vi "SMU Switch Handshaking - LV code improvements - Streaming2.vi"(8 "error in":errorcluster, 10 "gRPCid":T1, 11 "file path (use dialog)":path=path "C:/Users/IES/Desktop/jsontestfile.json") -> (0 "error out":errorcluster, 3 "Elapsed Time":u32)   [LabVIEW 2019]
uses:
  labview-grpc-query-server/VIs/MeasurementServer_gRPCid.ctl
  <instrlib>/niDCPower/nidcpower.llb/niDCPower Send Software Edge Trigger - Signal.ctl
  labview-grpc-query-server/VIs/MeasurementServer_FourProbeRawData.ctl
  labview-grpc-query-server/VIs/MeasurementServer_ErrorOutData.ctl
  <instrlib>/niDCPower/nidcpower.llb/niDCPower Configure Software Edge Start Trigger.vi
  <instrlib>/niDCPower/nidcpower.llb/niDCPower Configure Software Edge Sequence Advance Trigger.vi
  labview-grpc-query-server/VIs/labview-grpc-measurement-server.lvlib
  SupportVIs.lvlib
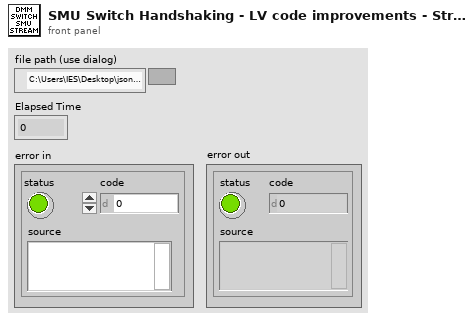
[diagram p1: front panel]
types:
  T1 = typedef "labview-grpc-measurement-server.lvlib/MeasurementServer_gRPCid.ctl" = u64
  T2 = typedef "niDCPower Send Software Edge Trigger - Signal.ctl" = i32
  T3 = typedef "JSONCluster.ctl" = cluster{"SMUResourceName":string, "SMUChannels":string, "SMUSourceMode_Sequence":i32, "SMUOutputFunction_DCCurrent":i32, "SMUSourceTransientResponse_Fast":i32, "SMUCurrent":dbl, "SMUCurrentLevelRange":dbl, "SMUMeasurementSense_Local":i32, "SMUMeasurementApertureTime":dbl, "SMUSourceAdvancedSourceDelay":dbl, "SMUVoltage":dbl, "SMUSourceAdvancedSequenceLoopCount":i32, "SMUMeasurementAdvancedDCNoiseRejection_Normal":i32, "SMUSequenceName":string, "SMUStep1_Source_DCCurrent_CurrentLevel":i32, "SMUStep2_Measurement_ApertureTime":i32, "SMUStep3_Source_Advanced_SourceDelay":i32, "SMUSequenceNumberOfSteps":i32, "SMUTriggerFromSwitch_StartDigitalEdge":string, "SMUTriggerFromSwitch_SequenceAdvanceDigitalEdge":string, "SMUTriggerToDMM_SourceCompleteEvent":i32, "SMUTriggerToDMM_SourceCompleteEvent_Value":string, "SMUTriggerToSwitch_SequenceIterationCompleteEvent":i32, "SMUTriggerToDMM_SequenceIterationCompleteEvent_Value":string, "Switch1ResourceName":string, "Switch1Topology":string, "Switch1ScanList":string, "Switch2ResourceName":string, "Switch2Topology":string, "Switch2ScanList":string, "DMMResourceName":string, "DMMFunction_DCVolts":i32, "DMMResolution":dbl, "DMMRange":dbl, "DMMTriggerSource_TTL2":i32, "DMMTriggerSlope_RisingEdge":i32, "DMMSampleTrigger_TTL2":i32, "DMMSampleCount":i32, "DMMSampleTriggerSlope_RisingEdge":i32, "DMMApertureTimeUnits_Seconds":i32, "DMMApertureTime":dbl, "DMMNumberOfAverages":i32, "DMMAutoZero_Off":i32, "DMMADCCalibration_Off":i32, "DMMSettleTime":dbl, "DMMControlAction_Commit":i32, "ApplicationNumberOfWeldChannels":i32}
  T4 = typedef "labview-grpc-measurement-server.lvlib/MeasurementServer_ErrorOutData.ctl" = cluster{"ErrorCode":i32, "ErrorMessage":string}
  T5 = typedef "labview-grpc-measurement-server.lvlib/MeasurementServer_FourProbeRawData.ctl" = cluster{"Positive Voltage":sgl, "Positive Current":sgl, "Negative Voltage":sgl, "Negative Current":sgl, "Impedance":sgl, "ErrorOutData":T4}
  T6 = typedef "niDMM Acquisition State.ctl" = enum16{"Running", "Finished with Backlog", "Finished with no Backlog", "Paused", "No acquisition in progress"}
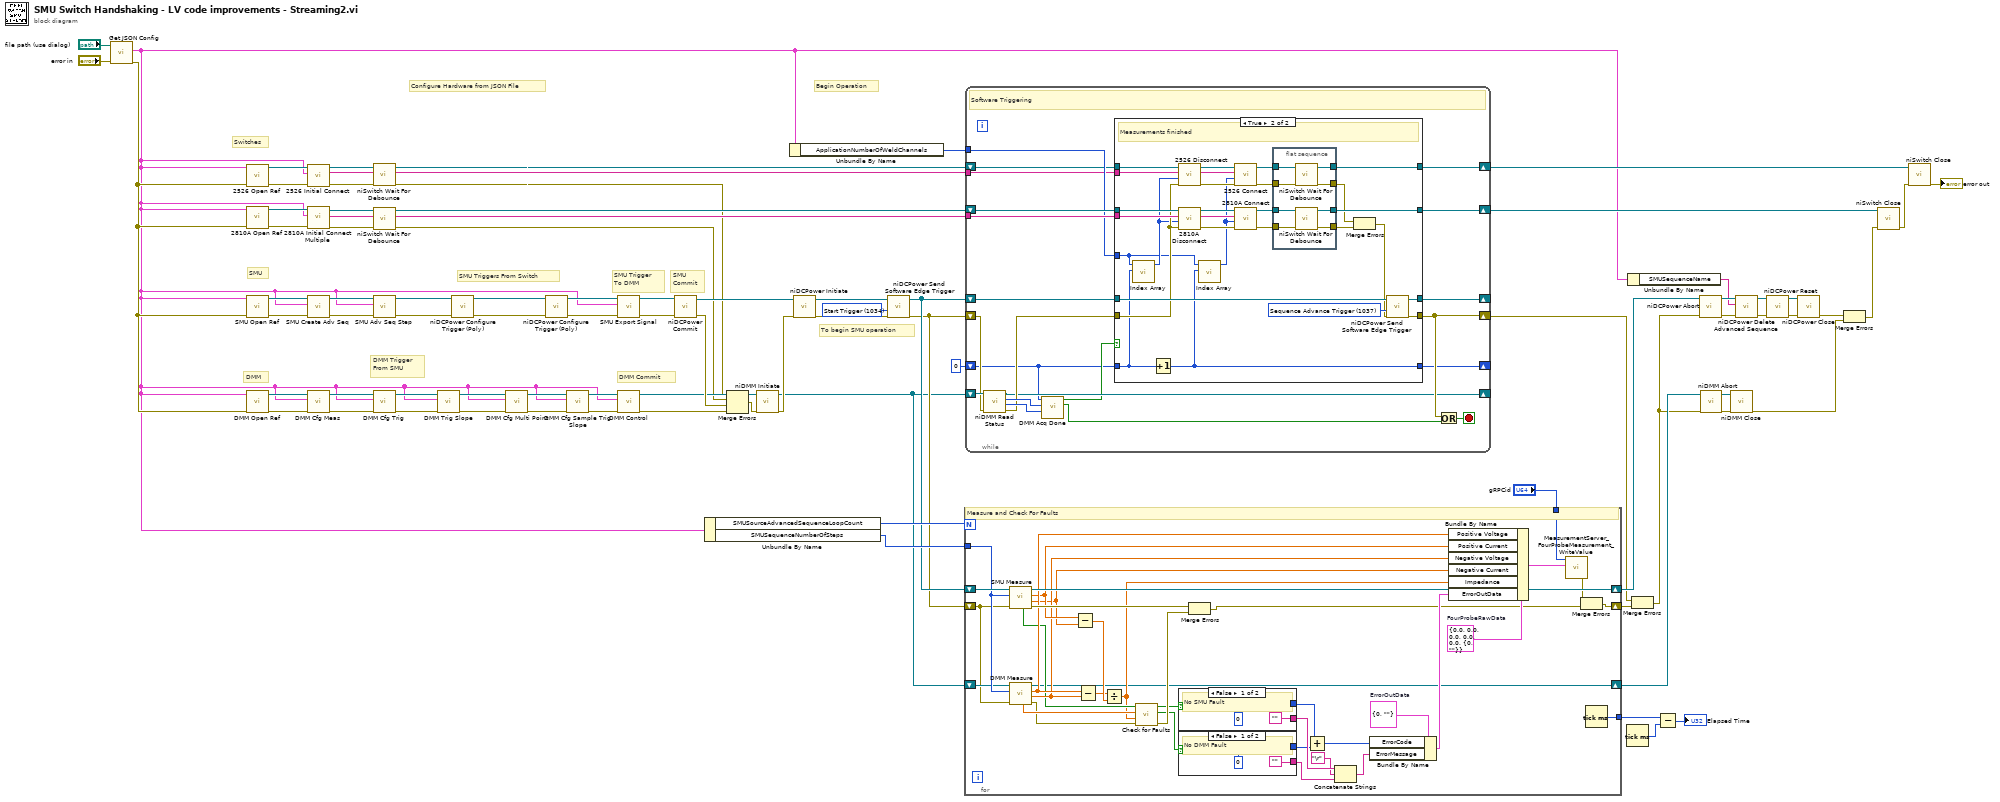
[diagram p0: block diagram]
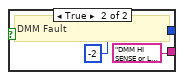
[diagram p3: hidden frame]
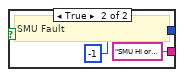
[diagram p4: hidden frame]
diagram:
  w35 = T2 1034 items=["Start Trigger"=1034, "Source Trigger"=1035, "Measure Trigger"=1036, "Sequence Advance Trigger"=1037, "Pulse Trigger"=1053] ("signal")
  # "SMU\nCommit"
  # "DMM Commit"
  # "Begin Operation"
  # "Configure Hardware from JSON File"
  # "DMM"
  # "SMU"
  # "Switches"
  # "To begin SMU operation"
  # "DMM Trigger\nFrom SMU"
  # "SMU Trigger \nTo DMM"
  # "SMU Triggers From Switch"
  n1 = call "Get JSON Config.vi"("error in (no error)"="error in", "JSON Configuration File (.json)"="file path (use dialog)") -> ("error out"=w9:errorcluster, "JSONCluster"=w2:T3)  [unwired: 6 in, 2 out]
  n2 = call "2526 Open Ref.vi"("error in"=w9, "JSONCluster"=w2) -> ("error out"=w21:errorcluster, "IVI Refnum out"=w22:refnum<k15>)  [unwired: 8 in]
  n3 = call "2810A Open Ref.vi"("error in"=w9, "JSONCluster"=w2) -> ("error out"=w28:errorcluster, "IVI Refnum out"=w29:refnum<k15>)  [unwired: 8 in]
  n4 = call "SMU Open Ref.vi"("error in (no error)"=w9, "JSONCluster"=w2) -> ("error out"=w82:errorcluster, "IVI Refnum out"=w83:refnum<k15>)  [unwired: 8 in]
  n5 = call "DMM Open Ref.vi"("error in"=w9, "JSONCluster"=w2) -> ("error out"=w55:errorcluster, "IVI Refnum out"=w54:refnum<k15>)  [unwired: 8 in]
  n6 = call "2526 Initial Connect.vi"("error in (no error)"=w21, "JSONCluster"=w2, "IVI Refnum in"=w22) -> ("error out"=w19:errorcluster, "2525 Scan List Channels"=w15:string[], "IVI Refnum out"=w20:refnum<k15>)  [unwired: 6 in]
  n7 = call "2810A Initial Connect Multiple.vi"("error in (no error)"=w28, "JSONCluster"=w2, "IVI Refnum in"=w29) -> ("error out"=w25:errorcluster, "Array"=w27:string[], "IVI Refnum out"=w26:refnum<k15>)  [unwired: 6 in]
  n8 = call "SMU Create Adv Seq.vi"("error in (no error)"=w82, "JSONCluster"=w2, "IVI Refnum in"=w83) -> ("error out"=w70:errorcluster, "IVI Refnum out"=w71:refnum<k15>)  [unwired: 7 in]
  n9 = call "DMM Cfg Meas.vi"("error in (no error)"=w55, "JSONCluster"=w2, "IVI Refnum in"=w54) -> ("error out"=w59:errorcluster, "IVI Refnum out"=w58:refnum<k15>)  [unwired: 7 in]
  n10 = call <instrlib>:"niSwitch Wait For Debounce.vi"("error in (no error)"=w19, "instrument handle"=w20) -> ("error out"=w17:errorcluster, "instrument handle out"=w16:refnum<k15>)  [unwired: 8 in]
  n11 = call <instrlib>:"niSwitch Wait For Debounce.vi"("error in (no error)"=w25, "instrument handle"=w26) -> ("error out"=w24:errorcluster, "instrument handle out"=w23:refnum<k15>)  [unwired: 8 in]
  n12 = call "SMU Adv Seq Step.vi"("error in (no error)"=w70, "JSONCluster"=w2, "IVI Refnum in"=w71) -> ("error out"=w68:errorcluster, "IVI Refnum out"=w69:refnum<k15>)  [unwired: 7 in]
  n13 = call "DMM Cfg Trig.vi"("error in (no error)"=w59, "JSONCluster"=w2, "IVI Refnum in"=w58) -> ("error out"=w61:errorcluster, "IVI Refnum out"=w60:refnum<k15>)  [unwired: 7 in]
  n14 = call "DMM Trig Slope.vi"("error in (no error)"=w61, "JSONCluster"=w2, "IVI Refnum in"=w60) -> ("error out"=w63:errorcluster, "IVI Refnum out"=w62:refnum<k15>)  [unwired: 7 in]
  n15 = call-poly <instrlib>:"niDCPower Configure Trigger (Poly).vi"("error in (no error)"=w68, "instrument handle"=w69) -> ("error out"=w79:errorcluster, "instrument handle out"=w80:refnum<k15>)  [unwired: 8 in]
  n16 = call "DMM Cfg Multi Point.vi"("error in (no error)"=w63, "JSONCluster"=w2, "IVI Refnum in"=w62) -> ("error out"=w65:errorcluster, "IVI Refnum out"=w64:refnum<k15>)  [unwired: 7 in]
  n17 = call-poly <instrlib>:"niDCPower Configure Trigger (Poly).vi"("error in (no error)"=w79, "instrument handle"=w80) -> ("error out"=w42:errorcluster, "instrument handle out"=w43:refnum<k15>)  [unwired: 8 in]
  n18 = call "DMM Cfg Sample Trig Slope.vi"("error in (no error)"=w65, "JSONCluster"=w2, "IVI Refnum in"=w64) -> ("error out"=w47:errorcluster, "IVI Refnum out"=w48:refnum<k15>)  [unwired: 7 in]
  n19 = call "SMU Export Signal.vi"("error in (no error)"=w42, "JSONCluster"=w2, "IVI Refnum in"=w43) -> ("error out"=w66:errorcluster, "IVI Refnum out"=w67:refnum<k15>)  [unwired: 7 in]
  n20 = call "DMM Control.vi"("error in (no error)"=w47, "JSONCluster"=w2, "IVI Refnum in"=w48) -> ("error out"=w52:errorcluster, "IVI Refnum out"=w49:refnum<k15>)  [unwired: 7 in]
  n21 = call <instrlib>:"niDCPower Commit.vi"("error in (no error)"=w66, "instrument handle"=w67) -> ("error out"=w53:errorcluster, "instrument handle out"=w50:refnum<k15>)  [unwired: 8 in]
  n22 = Unbundle By Name(w2) -> ("SMUSourceAdvancedSequenceLoopCount"=w38:i32, "SMUSequenceNumberOfSteps"=w37:i32)
  n23 = Merge Errors(w17, w24, w53, w52) -> (w51:errorcluster)
  n24 = call <instrlib>:"niDMM Initiate.vi"("error in (no error)"=w51, "instrument handle"=w49) -> ("error out"=w18:errorcluster, "instrument handle out"=w3:refnum<k15>)  [unwired: 8 in]
  n25 = Unbundle By Name(w2) -> ("ApplicationNumberOfWeldChannels"=w31:i32)
  n26 = call <instrlib>:"niDCPower Initiate.vi"("error in (no error)"=w18, "instrument handle"=w50) -> ("error out"=w30:errorcluster, "instrument handle out"=w36:refnum<k15>)  [unwired: 8 in]
  n27 = call <instrlib>:"niDCPower Send Software Edge Trigger.vi"("error in (no error)"=w30, "signal"=w35, "instrument handle"=w36) -> ("error out"=w4:errorcluster, "instrument handle out"=w5:refnum<k15>)  [unwired: 7 in]
  n28 = for {
    N: w38 -> [_]
    tunnel: w37 -> [w91]
    shift-right: [w89] -> w7
    shift-left: w4 -> [w87]
    shift-right: [w119] -> w81
    shift-left: w5 -> [w92]
    shift-right: [w85] -> w44
    shift-left: w3 -> [w88]
    tunnel: [w96] -> w10
    tunnel: "gRPCid" -> [w95]
    w97 = T4 {"ErrorCode"=0, "ErrorMessage"=""}  # ErrorOutData
    w94 = T5 {"Positive Voltage"=0.0, "Positive Current"=0.0, "Negative Voltage"=0.0, "Negative Current"=0.0, "Impedance"=0.0, "ErrorOutData"={"ErrorCode"=0, "ErrorMessage"=""}}  # FourProbeRawData
    # "Measure and Check For Faults"
    n29 = call "SMU Measure.vi"("error in (no error)"=w87, "SMUSequenceNumberOfSteps"=w91, "IVI Refnum in"=w92) -> ("error out"=w118:errorcluster, "Numeric"=w111:dbl, "Numeric 2"=w113:dbl, "IVI Refnum out"=w119:refnum<k15>, "in compliance"=w100:bool[])  [unwired: 4 in]
    n30 = call "DMM Measure.vi"("error in (no error)"=w87, "SMUSequenceNumberOfSteps"=w91, "IVI Refnum in"=w88) -> ("error out"=w86:errorcluster, "Numeric"=w112:dbl, "Numeric 2"=w114:dbl, "IVI Refnum out"=w85:refnum<k15>, "Measurements"=w99:dbl[])  [unwired: 4 in]
    n31 = Subtract(x=w113, y=w111) -> (x-y=w116:dbl)
    n32 = Subtract(x=w114, y=w112) -> (x-y=w115:dbl)
    n33 = Divide(x=w115, y=w116) -> (x/y=w98:dbl)
    n34 = call "Check for Faults.vi"("Error In"=w86, "Resistance In"=w98, "dmm voltage measurements"=w99, "in compliance"=w100) -> ("Error Out"=w117:errorcluster, "DMM Fault"=w104:bool, "SMU Fault"=w108:bool)  [unwired: 4 in, 1 out]
    n35 = case shown="False" w108 {
      tunnel: ["" "SMU HI or LO lead disconnected\n- SMU in compliance\n- SMU Fault = True"] -> w107
      tunnel: [0 -1] -> w105
      frame False {
        # "No SMU Fault"
      }
      frame True {
        # "SMU Fault"
      }
    }
    n36 = case shown="False" w104 {
      tunnel: ["" "DMM HI SENSE or LO SENSE lead disconnected\n- DMM measures NaN, or \n- DMM overrange warning, or\n- DMM voltage > 50uV "] -> w102
      tunnel: [0 -2] -> w101
      frame False {
        # "No DMM Fault"
      }
      frame True {
        # "DMM Fault"
      }
    }
    n37 = Merge Errors(w118, w117) -> (w84:errorcluster)
    n38 = Add(x=w105, y=w101) -> (x+y=w109:i32)
    n39 = Concatenate Strings(w107, "\r", w102) -> (w106:string)
    n40 = Bundle By Name(cluster=w97, "ErrorCode"=w109, "ErrorMessage"=w106) -> (w110:T4)
    n41 = Bundle By Name(cluster=w94, "Positive Voltage"=w114, "Positive Current"=w113, "Negative Voltage"=w112, "Negative Current"=w111, "Impedance"=w98, "ErrorOutData"=w110) -> (w93:T5)
    n42 = call "MeasurementServer_FourProbeMeasurement_WriteValue.vi"("gRPCid"=w95, "FourProbeRawData"=w93) -> ("error out"=w90:errorcluster)  [unwired: 8 in]
    n43 = Merge Errors(w90, w84) -> (w89:errorcluster)
    n44 = Tick Count (ms)() -> (millisecond timer value=w96:u32)
  }
  n45 = while {
    shift-right: [w148] -> _
    shift-left: w5 -> [w143]
    shift-right: [w146] -> w1
    shift-left: w4 -> [w133]
    shift-right: [w144] -> w32
    shift-left: w23 -> [w145]
    shift-right: [w131] -> _
    shift-left: w3 -> [w134]
    shift-right: [w142] -> _
    shift-left: 0 ("Backlog") -> [w128]
    tunnel: w27 -> [w141]
    tunnel: w31 -> [w140]
    shift-right: [w138] -> w14
    shift-left: w16 -> [w139]
    tunnel: w15 -> [w137]
    stop <- w147 stop-if-true
    # "Software Triggering"
    n46 = call <instrlib>:"niDMM Read Status.vi"("error in (no error)"=w133, "instrument handle"=w134) -> ("error out"=w132:errorcluster, "Acquisition State"=w135:T6, "Backlog"=w136:i32, "instrument handle out"=w131:refnum<k15>)  [unwired: 6 in]
    n47 = call "DMM Acq Done.vi"("Acquisition State"=w135, "Backlog"=w136, "Channel Index"=w128) -> ("Finished with Backlog?"=w129:bool, "Sequence Acquision Finished?"=w130:bool)  [unwired: 7 in]
    n48 = case shown="True" w130 {
      tunnel: w132 -> [w152 w162]
      tunnel: [w153 w180] -> w148
      tunnel: [w152 w179] -> w146
      tunnel: w143 -> [w153 w176]
      tunnel: w145 -> [w151 w175]
      tunnel: [w151 w178] -> w144
      tunnel: w128 -> [w150 w158]
      tunnel: [w150 w155] -> w142
      tunnel: w141 -> [_ w172]
      tunnel: w140 -> [_ w154]
      tunnel: w139 -> [w149 w167]
      tunnel: [w149 w164] -> w138
      tunnel: w137 -> [_ w163]
      frame False {
        # "Measurements not finished yet - repeat loop"
      }
      frame True {
        w177 = T2 1037 items=["Start Trigger"=1034, "Source Trigger"=1035, "Measure Trigger"=1036, "Sequence Advance Trigger"=1037, "Pulse Trigger"=1053] ("signal")
        # "Measurements finished"
        n49 = call "Index Array.vi"("Backlog"=w158, "ApplicationNumberOfWeldChannels"=w154) -> ("Index"=w157:i32)  [unwired: 9 in]
        n50 = Increment(x=w158) -> (x+1=w155:i32)
        n51 = call "2526 Disconnect.vi"("error in (no error)"=w162, "Index"=w157, "2525 Scan List Channels"=w163, "IVI Refnum in"=w167) -> ("error out"=w168:errorcluster, "IVI Refnum out"=w169:refnum<k15>)  [unwired: 6 in]
        n52 = call "2810A Disconnect.vi"("error in (no error)"=w162, "Numeric"=w157, "Array"=w172, "IVI Refnum in"=w175) -> ("error out"=w171:errorcluster, "IVI Refnum out"=w174:refnum<k15>)  [unwired: 6 in]
        n53 = call "Index Array.vi"("Backlog"=w155, "ApplicationNumberOfWeldChannels"=w154) -> ("Index"=w156:i32)  [unwired: 9 in]
        n54 = call "2526 Connect.vi"("error in (no error)"=w168, "Index"=w156, "2525 Scan List Channels"=w163, "IVI Refnum in"=w169) -> ("error out"=w165:errorcluster, "IVI Refnum out"=w166:refnum<k15>)  [unwired: 6 in]
        n55 = call "2810A Connect.vi"("error in (no error)"=w171, "Index"=w156, "Array"=w172, "IVI Refnum in"=w174) -> ("error out"=w170:errorcluster, "IVI Refnum out"=w173:refnum<k15>)  [unwired: 6 in]
        n56 = flat-sequence {
          tunnel: [w188] -> w178
          tunnel: [w187] -> w161
          tunnel: w173 -> [w186]
          tunnel: w170 -> [w185]
          tunnel: w166 -> [w184]
          tunnel: w165 -> [w183]
          tunnel: [w182] -> w164
          tunnel: [w181] -> w160
          frame #0 {
            n57 = call <instrlib>:"niSwitch Wait For Debounce.vi"("error in (no error)"=w183, "instrument handle"=w184) -> ("error out"=w181:errorcluster, "instrument handle out"=w182:refnum<k15>)  [unwired: 8 in]
            n58 = call <instrlib>:"niSwitch Wait For Debounce.vi"("error in (no error)"=w185, "instrument handle"=w186) -> ("error out"=w187:errorcluster, "instrument handle out"=w188:refnum<k15>)  [unwired: 8 in]
          }
        }
        n59 = Merge Errors(w160, w161) -> (w159:errorcluster)
        n60 = call <instrlib>:"niDCPower Send Software Edge Trigger.vi"("error in (no error)"=w159, "signal"=w177, "instrument handle"=w176) -> ("error out"=w179:errorcluster, "instrument handle out"=w180:refnum<k15>)  [unwired: 7 in]
      }
    }
    n61 = Or(x=w146, y=w129) -> (x .or. y?=w147:bool)
  }
  n62 = Tick Count (ms)() -> (millisecond timer value=w78:u32)
  n63 = Unbundle By Name(w2) -> ("SMUSequenceName"=w11:string)
  n64 = Merge Errors(w1, w7) -> (w6:errorcluster)
  n65 = Subtract(x=w10, y=w78) -> (x-y=→"Elapsed Time":u32)
  n66 = call <instrlib>:"niDCPower Abort.vi"("error in (no error)"=w6, "instrument handle"=w81) -> ("error out"=w76:errorcluster, "instrument handle out"=w77:refnum<k15>)  [unwired: 8 in]
  n67 = call <instrlib>:"niDMM Abort.vi"("error in (no error)"=w6, "instrument handle"=w44) -> ("error out"=w57:errorcluster, "instrument handle out"=w56:refnum<k15>)  [unwired: 8 in]
  n68 = call <instrlib>:"niDMM Close.vi"("error in (no error)"=w57, "instrument handle"=w56) -> ("error out"=w46:errorcluster)  [unwired: 9 in]
  n69 = call <instrlib>:"niDCPower Delete Advanced Sequence.vi"("error in (no error)"=w76, "sequence name"=w11, "instrument handle"=w77) -> ("error out"=w75:errorcluster, "instrument handle out"=w74:refnum<k15>)  [unwired: 7 in]
  n70 = call <instrlib>:"niDCPower Reset.vi"("error in (no error)"=w75, "instrument handle"=w74) -> ("error out"=w72:errorcluster, "instrument handle out"=w73:refnum<k15>)  [unwired: 2 in, 6 out]
  n71 = call <instrlib>:"niDCPower Close.vi"("error in (no error)"=w72, "instrument handle"=w73) -> ("error out"=w45:errorcluster)  [unwired: 9 in]
  n72 = Merge Errors(w45, w46) -> (w33:errorcluster)
  n73 = call <instrlib>:"niSwitch Close.vi"("error in (no error)"=w33, "instrument handle"=w32) -> ("error out"=w13:errorcluster)  [unwired: 9 out]
  n74 = call <instrlib>:"niSwitch Close.vi"("error in (no error)"=w13, "instrument handle"=w14) -> ("error out"=→"error out":errorcluster)  [unwired: 9 out]
